vi "Setup Trig.vi"(8 "Error IN":errorcluster, 10 "Trig Properties Ctl":T1, 11 "hCamera IN":u32) -> (0 "Error OUT":errorcluster, 3 "hCamera OUT":u32)   [LabVIEW 2014]
uses:
  Controls/Trig Properties.ctl
  <vilib>/addons/PixeLINK/Low Level Functions/CAMERA_FEATURES.llb/TDPU-CameraFeatures-FeatureFlags.ctl
  <vilib>/addons/PixeLINK/Low Level Functions/CAMERA_FEATURES.llb/TDPU-CameraFeatures-FeatureIds.ctl
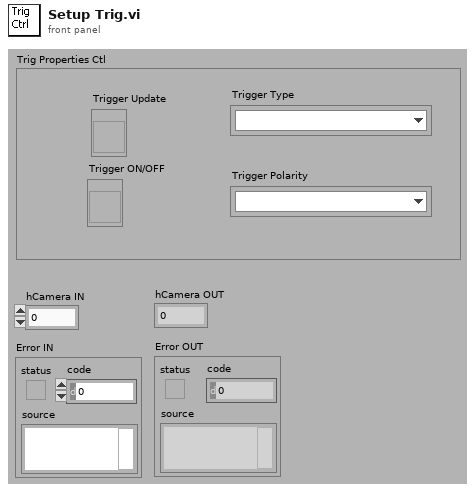
[diagram p1: front panel]
types:
  T1 = typedef "Trig Properties.ctl" = cluster{"Trigger ON/OFF":refnum<vi>, "Trigger Type":refnum<vi>, "Trigger Polarity":refnum<vi>, "Trigger Update":refnum<vi>}
  T2 = typedef "TDPU-CameraFeatures-FeatureIds.ctl" = u32
  T3 = typedef "TDPU-CameraFeatures-FeatureFlags.ctl" = u32
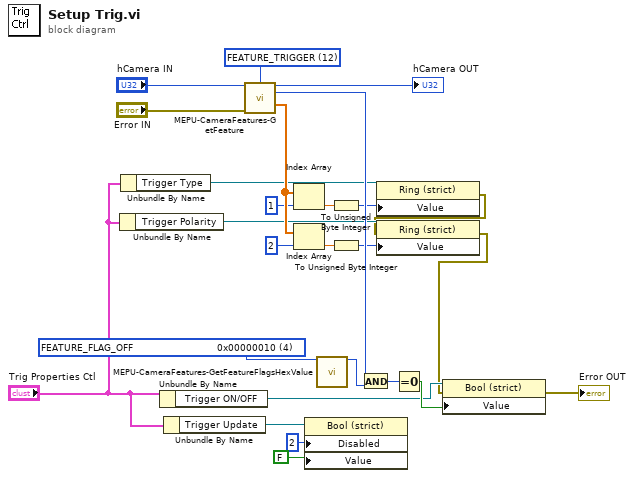
[diagram p0: block diagram]
diagram:
  w18 = T2 12 items=["FEATURE_BRIGHTNESS", "FEATURE_EXPOSURE", "FEATURE_SHARPNESS", "FEATURE_WHITE_BAL", "FEATURE_HUE", "FEATURE_SATURATION", "FEATURE_GAMMA", "FEATURE_SHUTTER", "FEATURE_GAIN", "FEATURE_IRIS", "FEATURE_FOCUS", "FEATURE_TEMPERATURE", "FEATURE_TRIGGER", "FEATURE_ZOOM", "FEATURE_PAN", "FEATURE_TILT", "FEATURE_OPT_FILTER", "FEATURE_GPIO", "FEATURE_FRAME_RATE", "FEATURE_ROI", "FEATURE_FLIP", "FEATURE_DECIMATION", "FEATURE_PIXEL_FORMAT", "FEATURE_EXTENDED_SHUTTER", "FEATURE_AUTO_ROI", "FEATURE_LOOKUP_TABLE", "FEATURE_MEMORY_CHANNEL", "FEATURE_ALL"] ("uFeatureId IN")
  w3 = T3 4 items=["FEATURE_FLAG_PRESENCE                 0x00000001", "FEATURE_FLAG_MANUAL                     0x00000002", "FEATURE_FLAG_AUTO                         0x00000004", "FEATURE_FLAG_ONEPUSH                   0x00000008", "FEATURE_FLAG_OFF                            0x00000010", "FEATURE_FLAG_DESC_SUPPORTED    0x00000020", "FEATURE_FLAG_READ_ONLY               0x00000040"] ("uFlags OUT")
  n1 = Unbundle By Name("Trig Properties Ctl") -> ("Trigger Polarity"=w12:refnum<vi>)
  n2 = Unbundle By Name("Trig Properties Ctl") -> ("Trigger Type"=w13:refnum<vi>)
  n3 = Unbundle By Name("Trig Properties Ctl") -> ("Trigger ON/OFF"=w14:refnum<vi>)
  n4 = Unbundle By Name("Trig Properties Ctl") -> ("Trigger Update"=w7:refnum<vi>)
  n5 = call <vilib>:"MEPU-CameraFeatures-GetFeature.vi"("hCamera IN"="hCamera IN", "uFeatureId IN"=w18, "Error IN"="Error IN") -> ("hCamera OUT"=→"hCamera OUT":u32, "uFlags OUT"=w24:T3, "pParms OUT"=w23:dbl[])  [unwired: 1 in, 9 out]
  n6 = Index Array(array=w23, index=1) -> (element=w20:dbl)
  n7 = Index Array(array=w23, index=2) -> (element=w22:dbl)
  n8 = property class="Bool (strict)"(reference=w7, "Disabled"=u8 2, "Value"=FALSE) -> ()  [unwired: 1 in, 2 out]
  n9 = call <vilib>:"MEPU-CameraFeatures-GetFeatureFlagsHexValue.vi"("FeatureFlags"=w3) -> ("HexValue OUT"=w2:i32)  [unwired: 1 in, 13 out]
  n10 = To Unsigned Byte Integer(number=w20) -> (unsigned 8bit integer=w11:u8)
  n11 = To Unsigned Byte Integer(number=w22) -> (unsigned 8bit integer=w10:u8)
  n12 = And(x=w24, y=w2) -> (x .and. y?=w25:T3)
  n13 = property class="Ring (strict)"(reference=w13, "Value"=w11) -> (error out=w9:errorcluster)  [unwired: 1 in, 1 out]
  n14 = property class="Ring (strict)"(reference=w12, error in=w9, "Value"=w10) -> (error out=w1:errorcluster)  [unwired: 1 out]
  n15 = Equal To 0?(x=w25) -> (x = 0?=w26:bool)
  n16 = property class="Bool (strict)"(reference=w14, error in=w1, "Value"=w26) -> (error out=→"Error OUT":errorcluster)  [unwired: 1 out]
